vi "Queue Comms Enqueue.vi"(6 "Priority (F)":bool, 8 "error in (no error)":errorcluster, 10 "Element":T1) -> (0 "error out":errorcluster)   [LabVIEW 2020, in "Controller.lvlib"]
uses:
  Controller.lvlib
  Private Controls/Element.ctl
  Private Controls/Module Action.ctl
  Queue FGV Action.ctl
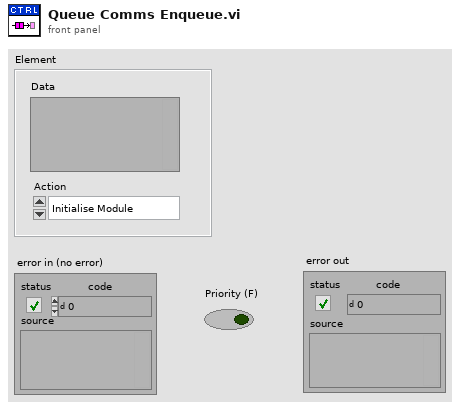
[diagram p1: front panel]
types:
  T1 = typedef "Controller.lvlib/Element.ctl" = cluster{"Action":T2, "Data":variant}
  T2 = typedef "Controller.lvlib/Module Action.ctl" = enum16{"Initialise Module", "Connect", "Setup", "Pause", "Start", "Search Network", "Get Local", "Stop", "Wait: Time Elapsed", "Error", "Exit"}
  T3 = typedef "Controller.lvlib/Queue FGV Action.ctl" = enum16{"Get", "Set", "Release"}
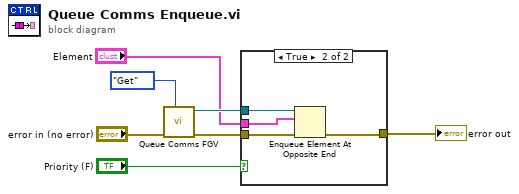
[diagram p0: block diagram]
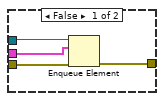
[diagram p2: hidden frame]
diagram:
  n1 = call "Queue Comms FGV.vi"("Action"=Queue_FGV_Action."Get", "error in (no error)"="error in (no error)") -> ("error out"=w5:errorcluster, "queue In"=w2:refnum<queue>)  [unwired: 8 in]
  n2 = case shown="True" "Priority (F)" {
    tunnel: w5 -> [w11 w15]
    tunnel: [w10 w14] -> w4
    tunnel: w2 -> [w9 w13]
    tunnel: "Element" -> [w8 w12]
    frame False {
      n3 = Enqueue Element(queue=w9, element=w8, error in (no error)=w11) -> (error out=w10:errorcluster)  [unwired: 1 in, 2 out]
    }
    frame True {
      n4 = Enqueue Element At Opposite End(queue=w13, element=w12, error in (no error)=w15) -> (error out=w14:errorcluster)  [unwired: 1 in, 2 out]
    }
  }
  "error out" <- w4
